vi "workspace.get_all.vi"(8 "error in":errorcluster, 11 "Nominal Client in":refnum<class "Nominal Client.lvclass">) -> (0 "error out":errorcluster, 2 "Workspaces":refnum<class "workspace.lvclass">[](array[class]), 3 "Nominal Client out":refnum<class "Nominal Client.lvclass">)   [LabVIEW 2020, in "Nominal Client.lvclass"]
doc: "Gets all workspaces that the requesting user belongs to."
uses:
  Nominal Client.lvclass
  nominal types/workspace/workspace.lvclass
  Nominal Client.lvclass/Nominal Client.ctl
  create.authorization_header.vi
  trace.payload_sent.vi
  trace.payload_received.vi
  error.vi
  api_token.get.vi
  error.vi/859f8e04-e495-489b-b5b4-7ac163f56130.vi
  submodules/reqwest-labview/lv-src/reqwest/get.vi
  <vilib>/JDP Science/JSONtext/Get all Object Items.vi
  <vilib>/Utility/error.llb/Error Cluster From Error Code.vi
  <vilib>/JDP Science/JSONtext/JSON text to Variant.vi
  <vilib>/JDP Science/JSONtext/LVClass Serializer/JSONtext LVClass Serializer.lvclass
  <vilib>/JDP Science/JSONtext/JSONtext.lvlib
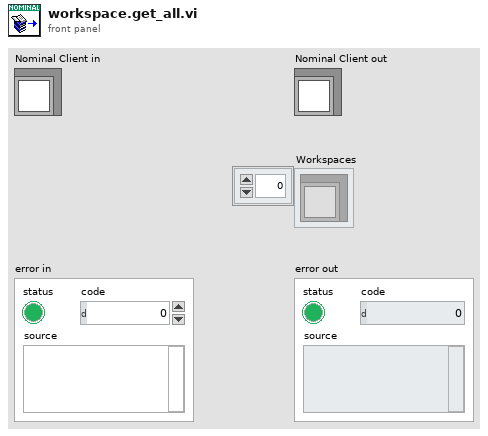
[diagram p1: front panel]
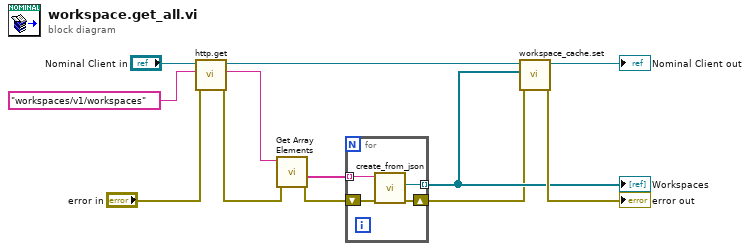
[diagram p0: block diagram]
diagram:
  n1 = call "http.get.vi"("error in"="error in", "Path"="workspaces/v1/workspaces", "Nominal Client in"="Nominal Client in") -> ("error out"=w1:errorcluster, "Response"=w6:string, "Nominal Client out"=w9:refnum<class "Nominal Client.lvclass">)  [unwired: 6 in]
  n2 = call <vilib>:"Get Array Elements.vi"("error in (no error)"=w1, "JSON"=w6) -> ("error out"=w3:errorcluster, "<JSON>"=w5:string[])  [unwired: 7 in, 1 out]
  n3 = for {
    tunnel: w5 -> [w16] mode=indexing
    tunnel: [w15] -> w4 mode=indexing
    shift-right: [w13] -> w2
    shift-left: w3 -> [w14]
    n4 = call "create_from_json.vi"("error in"=w14, "JSON"=w16) -> ("error out"=w13:errorcluster, "Workspace"=w15:refnum<class "workspace.lvclass">)  [unwired: 8 in]
  }
  "Workspaces" <- w4
  n5 = call "workspace_cache.set.vi"("error in"=w2, "Available Workspaces"=w4, "Nominal Client in"=w9) -> ("error out"=→"error out":errorcluster, "Nominal Client out"=→"Nominal Client out":refnum<class "Nominal Client.lvclass">)  [unwired: 7 in]
